vi "BIN_PAQ_decompose_chunk.vi"(8 "error in (no error)":errorcluster, 9 "Offset":cluster{"Offset":u32, "Size":u32}, 11 "Content":string) -> (0 "error out":errorcluster, 1 "Samples size":i32, 3 "PAQ_data":T1)   [LabVIEW 2020, in "Sgraph_lib_V1.lvlib" / "DBAL-BIN.lvclass"]
doc: "Decompose a file content chunck into an array with PAQ samples"
uses:
  DBAL-BIN.lvclass
  controls/BIN/BINdata.ctl
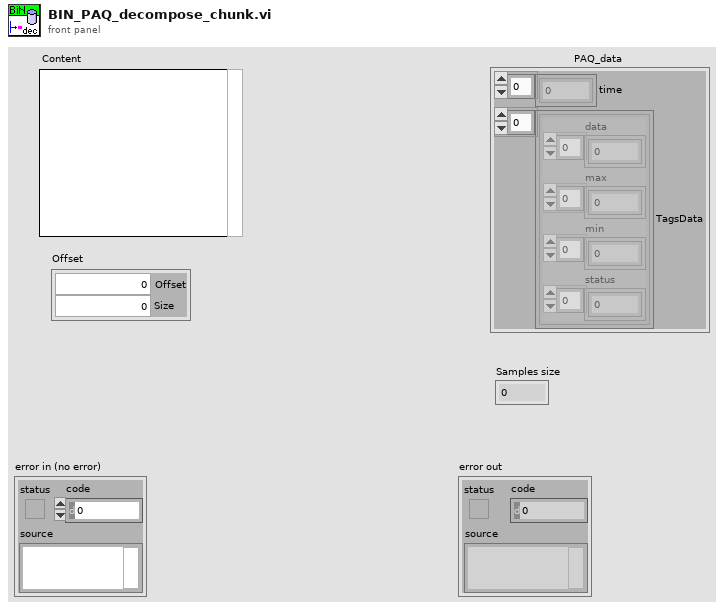
[diagram p1: front panel]
types:
  T1 = typedef "Sgraph_lib_V1.lvlib/DBAL-BIN.lvclass/BINdata.ctl" = cluster{"time":dbl[], "TagsData":cluster{"data":dbl[], "max":dbl[], "min":dbl[], "status":u32[]}[]}
  T2 = enum16{"big-endian, network order", "native, host order", "little-endian"}
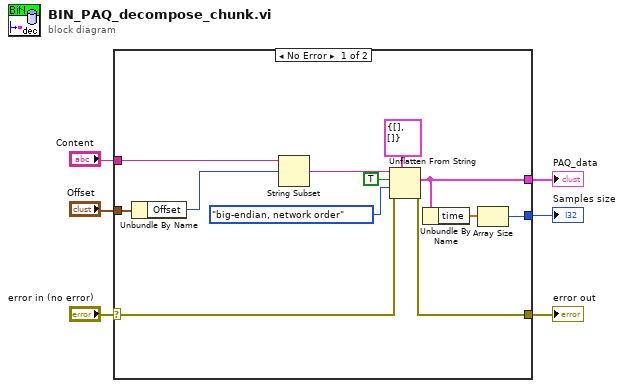
[diagram p0: block diagram]
diagram:
  n1 = case shown="No Error" "error in (no error)" {
    selector: "error in (no error)" -> [w10 w19]
    tunnel: [w9 w19] -> w5
    tunnel: "Content" -> [w12 _]
    tunnel: "Offset" -> [w11 _]
    tunnel: [w8 _] -> w2
    tunnel: [w7 _] -> w1
    frame No Error {
      n2 = Unbundle By Name(w11) -> ("Offset"=w18:u32)
      n3 = String Subset(string=w12, offset (0)=w18) -> (substring=w17:string)  [unwired: 1 in]
      n4 = Unflatten From String(type=T1 {"time"=[], "TagsData"=[]} ("BinHistData"), binary string=w17, data includes array or string size? (T)=TRUE, byte order (0:big-endian, network order)=T2."big-endian, network order", error in (no error)=w10) -> (value=w8:T1, error out=w9:errorcluster)  [unwired: 1 out]
      n5 = Unbundle By Name(w8) -> ("time"=w13:dbl[])
      n6 = Array Size(array=w13) -> (size(s)=w7:i32)
    }
    frame Error {
    }
  }
  "error out" <- w5
  "PAQ_data" <- w2
  "Samples size" <- w1
